vi "host.vi"() -> ()   [LabVIEW 2020]
uses:
  <vilib>/FPGAPlugInAG/cRIO-9035/niLvFpga_Open_cRIO-9035.vi
  <vilib>/rvi/interface/common/dynamic/niFpgaDynamicAddResources.vi
  <vilib>/Utility/error.llb/Error Cluster From Error Code.vi
  <vilib>/rvi/errors/niLvFpgaAdjustHostInterfaceError.vi
  <vilib>/FPGAPlugInAG/Dynamic/niLvFpga_Run_Dynamic.vi
  <vilib>/FPGAPlugInAG/Dynamic/niLvFpga_Close_Dynamic.vi
  <vilib>/rvi/interface/nirviOpenFPGA/nirviOpenFPGA.xnode
  FPGA Bitfiles/fftfpgaapplicati_FPGATarget_FFT2_NwCtSfbxiqQ.lvbitx
  FFT.vi
  <vilib>/rvi/interface/nirviMethod/nirviMethod.xnode
  <vilib>/rvi/interface/nirviCloseFPGA/nirviCloseFPGA.xnode
  <vilib>/rvi/errors/niLvFpgaMergeErrorWithErrorCode.vi
  <vilib>/FPGAPlugInAG/Dynamic/niLvFpga_ReadFifo_Dynamic.vi
  <vilib>/rvi/Analysis/host/Public/NI_FpgaMspHost.lvlib
  <vilib>/ptbypt/NI_PtbyPt.lvlib
  <vilib>/Analysis/NI_AALPro.lvlib
  <vilib>/FPGAPlugInAG/Dynamic/niLvFpga_WriteFifo_Dynamic.vi
panel:
  out "real size":i32
  out "img size":i32
  out "imaginary":dbl[](array[numeric])
  out "real":dbl[](array[numeric])
  out "imaginary number":dbl[](array[numeric])
  out "real number":dbl[](array[numeric])
  out "truth vs prediction vs error":dbl[][](graph)
  out "detrend acc":dbl[](graph)
  out "Array 3":dbl[](array[numeric])
  out "all rows":dbl[](array[numeric])
  out "XY Graph 2":cluster{dbl[], dbl[]}(graph)
  out "magnitude 2":dbl[](array[numeric])
  out "phase 2":dbl[](array[numeric])
  out "ploted signal from each selected frequency 2":dbl[][](graph)
  out "phase 1":dbl[](array[numeric])
  out "mag 1":dbl[](array[numeric])
  out "df (Hz) 2":dbl
  out "after FFT samples":i32
  out "xf (frequency)":dbl[](array[numeric])
  out "Before FFT samples":i32
  out "acc":dbl[](graph)
  out "samples":i32
  out "Array":fxp<+/-,32,16>[](array[numeric])
  out "end tick":fxp<+/-,32,16>[](array[numeric])
  out "start ticka":fxp<+/-,32,16>[](array[numeric])
  out "Waveform Graph":dbl[][](graph)
  out "input signal":T1(graph)
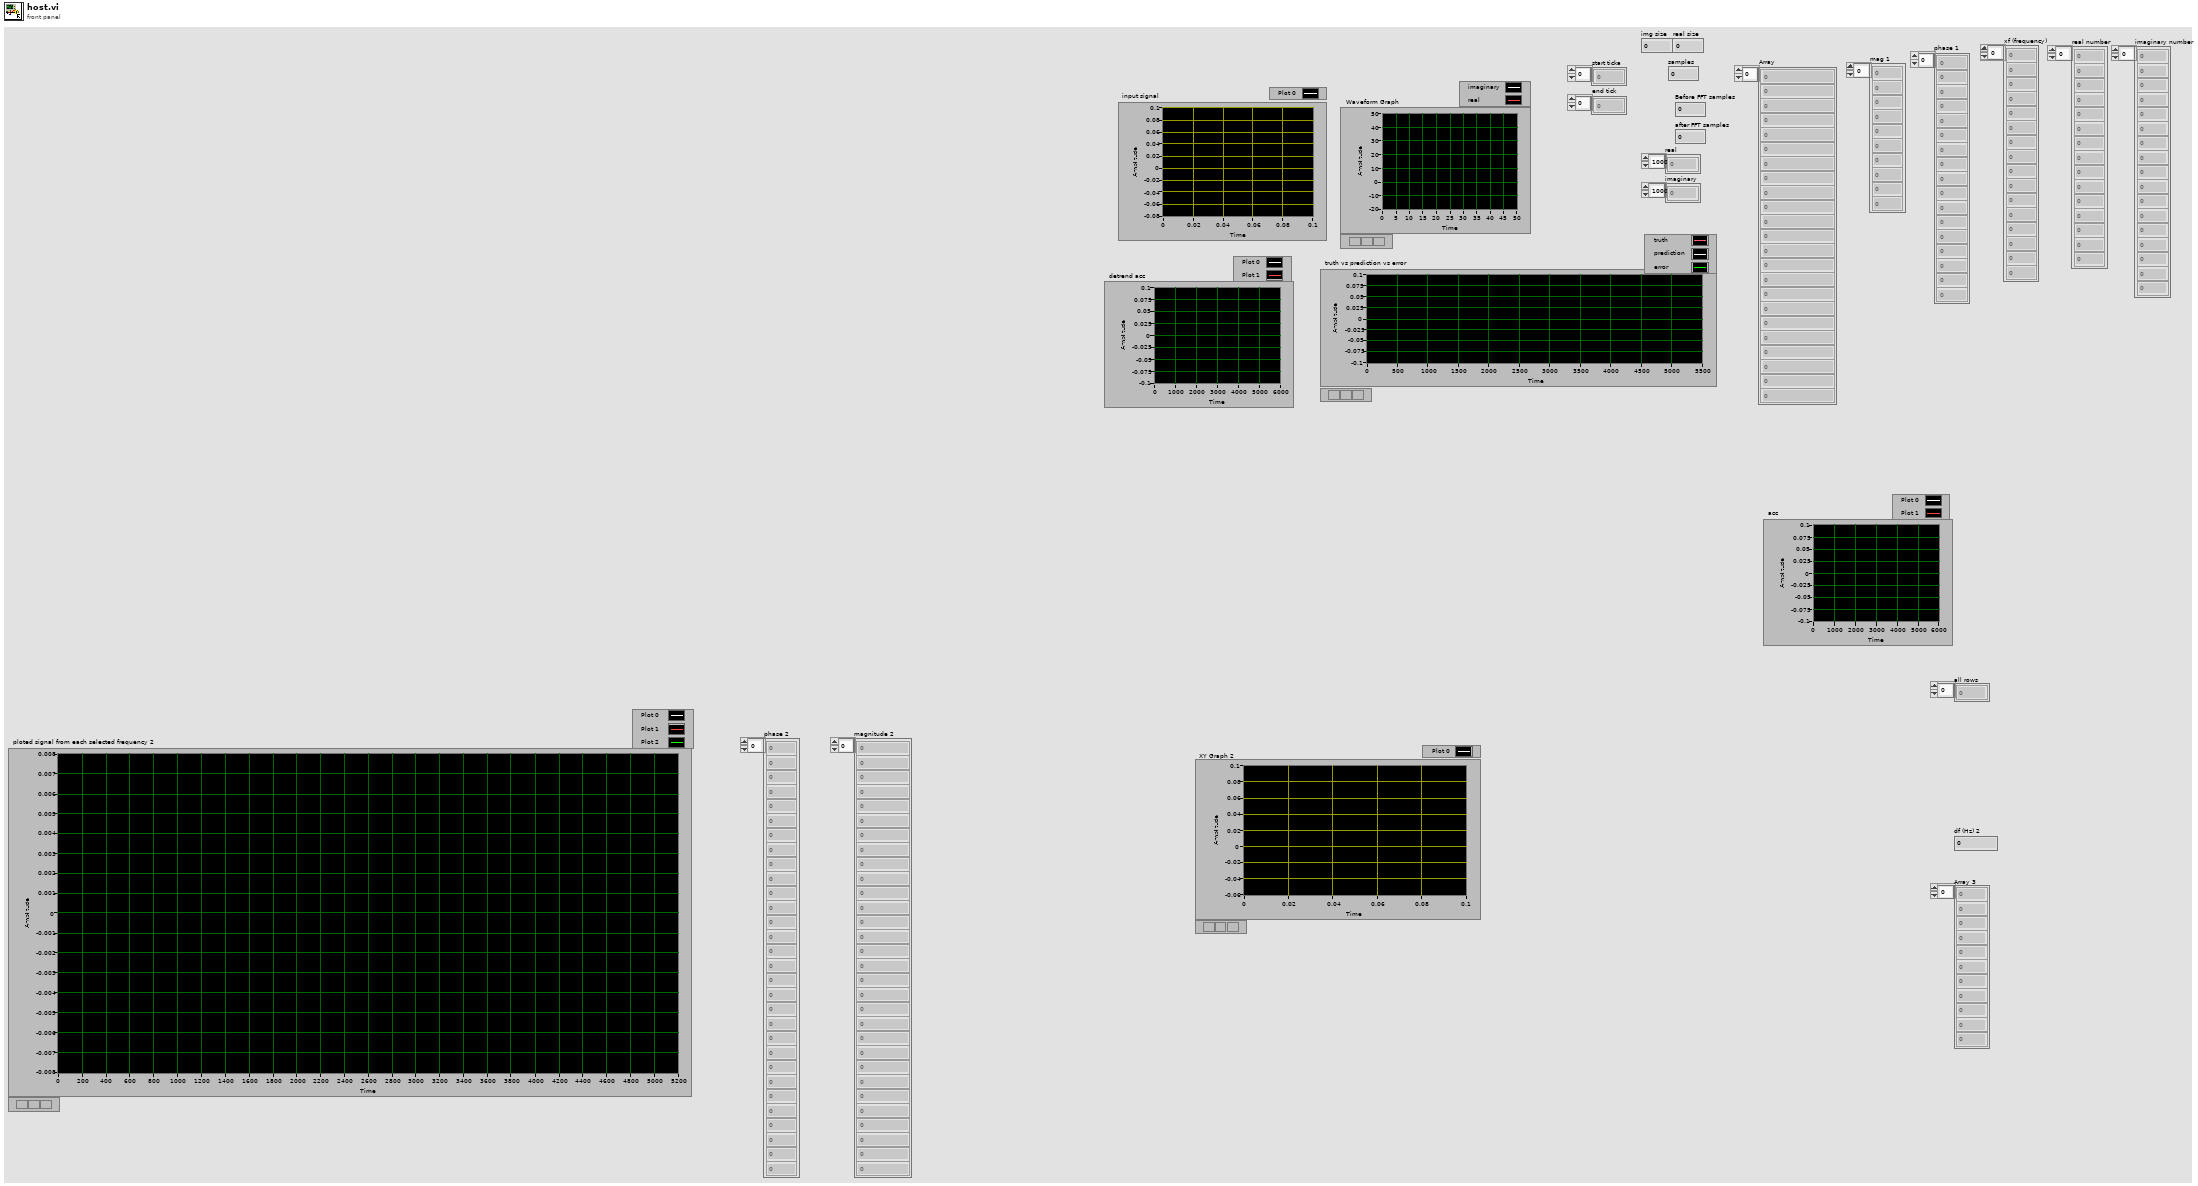
[diagram p1: front panel]
types:
  T1 = cluster{"array type (2D Dbl)":dbl[], "array type (2D Dbl)":dbl[]}
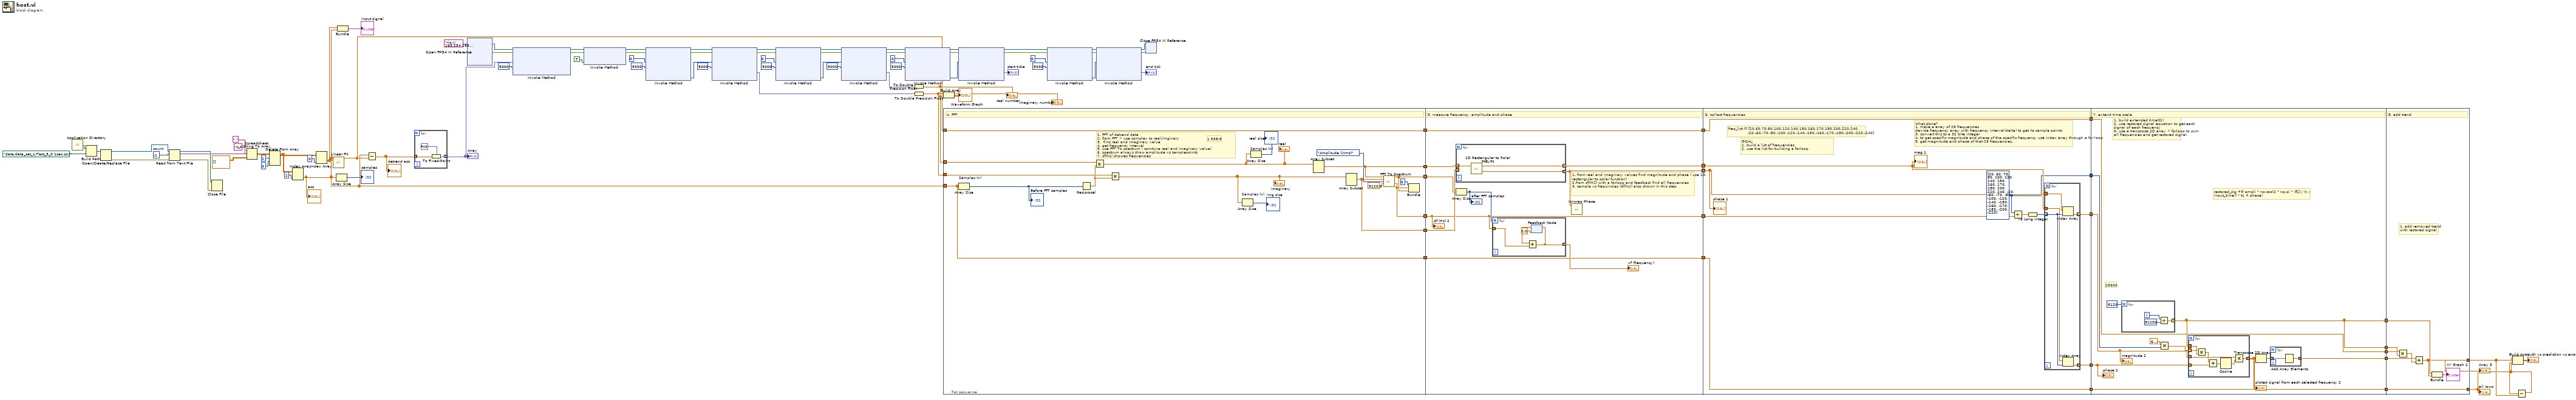
[diagram p0: block diagram]
diagram:
  w87 = -1  # count
  n1 = call <vilib>:"Application Directory.vi"() -> ("Application Directory"=w91:path)
  n2 = Build Path(base path=w91, name or relative path=path "data/data_set_1/Test_5_0.1sec.csv" ("default name")) -> (appended path=w90:path)
  n3 = Open/Create/Replace File(file path (use dialog)=w90) -> (refnum out=w95:refnum<file>, error out=w96:errorcluster)  [unwired: 5 in, 1 out]
  n4 = Read from Text File(file (use dialog)=w95, count=w87, error in=w96) -> (refnum out=w94:refnum<file>, text=w92:string, error out=w93:errorcluster)  [unwired: 1 in, 1 out]
  n5 = Close File(refnum=w94, error in=w93) -> ()  [unwired: 2 out]
  n6 = Spreadsheet String To Array(delimiter (Tab)=",", format string="%f", spreadsheet string=w92, array type (2D Dbl)=dbl[][] []) -> (array=w84:dbl[][])
  n7 = Delete From Array(array=w84, length=1, index (row)=0) -> (array with subset deleted=w79:dbl[][])  [unwired: 1 in, 1 out]
  n8 = Index Array(array=w79, index (col)=1 ("disabled index (col)")) -> (element=w6:dbl[])  [unwired: 1 in]
  "acc" <- w6
  n9 = Index Array(array=w79, index (col)=0 ("disabled index (col)")) -> (element=w10:dbl[])  [unwired: 1 in]
  n10 = call <vilib>:"Linear Fit.vi"("Y"=w6, "X"=w10) -> ("Best Linear Fit"=w7:dbl[])  [unwired: 9 in, 4 out]
  n11 = Array Size(array=w6) -> (size(s)=→"samples":i32)
  n12 = Bundle("array type (2D Dbl)"=w10, "array type (2D Dbl)"=w6) -> (→"input signal":T1)  [unwired: 1 in]
  n13 = Subtract(x=w6, y=w7) -> (x-y=w8:dbl[])
  "detrend acc" <- w8
  n14 = for {
    tunnel: [w98] -> w33 mode=indexing
    tunnel: w8 -> [w97] mode=indexing
    n15 = To Fixed-Point(fixed-point type=fxp<+/-,32,16> 0.0 ("f"), number=w97) -> (fixed-point=w98:fxp<+/-,32,16>)
  }
  "Array" <- w33
  n16 = xnode "Open FPGA VI Reference"("resource name"=tag "rio://169.254.183.73/RIO0") -> ("FPGA VI Reference Out"=w77:refnum<k20>, "error out"=w76:errorcluster)  [unwired: 1 in]
  n17 = xnode "Invoke Method"("FPGA VI Reference In"=w77, "error in"=w76, "Data"=w33, "Timeout (ms)"=5000) -> ("FPGA VI Reference Out"=w74:refnum<k20>, "error out"=w73:errorcluster)  [unwired: 1 out]
  n18 = xnode "Invoke Method"("FPGA VI Reference In"=w74, "error in"=w73, "Wait Until Done (F)"=TRUE) -> ("FPGA VI Reference Out"=w72:refnum<k20>, "error out"=w71:errorcluster)
  n19 = xnode "Invoke Method"("FPGA VI Reference In"=w72, "error in"=w71, "Number of Elements"=u32 0, "Timeout (ms)"=5000) -> ("FPGA VI Reference Out"=w70:refnum<k20>, "error out"=w69:errorcluster, "Elements Remaining"=w63:u32)  [unwired: 1 out]
  n20 = xnode "Invoke Method"("FPGA VI Reference In"=w70, "error in"=w69, "Number of Elements"=w63, "Timeout (ms)"=5000) -> ("FPGA VI Reference Out"=w66:refnum<k20>, "error out"=w65:errorcluster, "Data"=w60:fxp<+/-,32,16>[])  [unwired: 1 out]
  n21 = xnode "Invoke Method"("FPGA VI Reference In"=w66, "error in"=w65, "Number of Elements"=u32 0, "Timeout (ms)"=5000) -> ("FPGA VI Reference Out"=w68:refnum<k20>, "error out"=w67:errorcluster, "Elements Remaining"=w61:u32)  [unwired: 1 out]
  n22 = xnode "Invoke Method"("FPGA VI Reference In"=w68, "error in"=w67, "Number of Elements"=w61, "Timeout (ms)"=5000) -> ("FPGA VI Reference Out"=w56:refnum<k20>, "error out"=w55:errorcluster, "Data"=w59:fxp<+/-,32,16>[])  [unwired: 1 out]
  n23 = xnode "Invoke Method"("FPGA VI Reference In"=w56, "error in"=w55, "Number of Elements"=u32 0, "Timeout (ms)"=5000) -> ("FPGA VI Reference Out"=w54:refnum<k20>, "error out"=w53:errorcluster, "Elements Remaining"=w46:u32)  [unwired: 1 out]
  n24 = To Double Precision Float(number=w59) -> (double precision float=w5:dbl[])
  "real number" <- w5
  n25 = To Double Precision Float(number=w60) -> (double precision float=w9:dbl[])
  "imaginary number" <- w9
  n26 = Build Array(w9, w5) -> (→"Waveform Graph":dbl[][])
  n27 = flat-sequence {
    tunnel: [w115] -> w31
    tunnel: [w105] -> w30
    tunnel: [w104] -> w29
    tunnel: [w111] -> w28
    tunnel: [w110] -> w27
    tunnel: [w109] -> w26
    tunnel: w9 -> [w107]
    tunnel: w7 -> [w110]
    tunnel: w6 -> [w109]
    tunnel: w5 -> [w106]
    tunnel: w31 -> [w126]
    tunnel: w30 -> [w125]
    tunnel: w29 -> [w121]
    tunnel: w28 -> [w123]
    tunnel: [w121] -> w25
    tunnel: [w120] -> w24
    tunnel: [w119] -> w23
    tunnel: [w118] -> w22
    tunnel: w27 -> [w118]
    tunnel: w26 -> [w117]
    tunnel: [w117] -> w21
    tunnel: w25 -> [w135]
    tunnel: [w141] -> w20
    tunnel: w24 -> [w140]
    tunnel: w23 -> [w139]
    tunnel: [w138] -> w19
    tunnel: [w134] -> w18
    tunnel: [w137] -> w17
    tunnel: w22 -> [w137]
    tunnel: w21 -> [w136]
    tunnel: [w136] -> w16
    tunnel: w20 -> [w158]
    tunnel: w19 -> [w159]
    tunnel: w18 -> [w154]
    tunnel: [w152] -> w15
    tunnel: [w151] -> w14
    tunnel: w17 -> [w151]
    tunnel: [w150] -> w13
    tunnel: [w150] -> w12
    tunnel: w16 -> [w149]
    tunnel: [w149] -> w11
    tunnel: w15 -> [w181]
    tunnel: w14 -> [w179]
    tunnel: w13 -> [w180]
    tunnel: w12 -> [w178]
    tunnel: [w177] -> w2
    tunnel: w11 -> [w177]
    tunnel: [w176] -> w3
    frame #0 {
      # "1.95E-5"
      # "1. FFT of detrend data\n2. from FFT > use complex to real/imginary\n3.  find real and imaginary value\n4. get frequency interval\n5. use FFT To spectrum ( combine real and imaginary value)\n6. spectrum always show amplitude vs samplepoints\n7. df(hz) showes frequencies"
      # "4. FFT"
      n28 = Array Size "Samples (n)"(array=w109) -> (size(s)=w113:i32)
      "Before FFT samples" <- w113
      n29 = Reciprocal(x=w113) -> (1/x=w116:dbl)
      n30 = Multiply(x=w106, y=w116) -> (x*y=w101:dbl[])
      "real" <- w101
      n31 = Multiply(x=w107, y=w116) -> (x*y=w103:dbl[])
      "imaginary" <- w103
      n32 = Array Size "Samples (n)"(array=w103) -> (size(s)=→"img size":i32)
      n33 = Array Size "Samples (n)"(array=w101) -> (size(s)=→"real size":i32)
      n34 = Array Subset(array=w101) -> (w115:dbl[])  [unwired: 2 in]
      n35 = Array Subset(array=w103) -> (w105:dbl[])  [unwired: 2 in]
      n36 = call <vilib>:"FFT To Spectrum.vi"("real FFT data"=w115, "imaginary FFT data"=w105, "spectrum type"=enum8{"Power (Vrms^2)", "Amplitude (Vrms)"}."Amplitude (Vrms)", "sample rate (S/s)"=5120.0) -> ("spectrum out"=w111:dbl[], "df (Hz)"=w104:dbl)  [unwired: 9 in, 1 out]
      n37 = Bundle("index (row)"=0, "df (Hz)"=w104, "spectrum out"=w111) -> ()  [unwired: 1 in, 1 out]
    }
    frame #1 {
      # "1. from real and imaginary values find magnitude and phase ( use 1D rectangular to polar function)\n2.from df(HZ) with a forloop and feedback find all frequencies \n3. sample vs frequincies (df(hz)) also shown in this step"
      # "5. measure frequency, amplitude and phase"
      n38 = for {
        tunnel: w126 -> [w133] mode=indexing
        tunnel: w125 -> [_] mode=indexing
        tunnel: [w131] -> w120 mode=indexing
        tunnel: [w132] -> w119 mode=indexing
        n39 = call <vilib>:"1D Rectangular to Polar PtByPt.vi"("x"=w133) -> ("phase"=w132:dbl, "magnitude"=w131:dbl)  [unwired: 1 in]
      }
      n40 = Array Size(array=w123) -> (size(s)=w124:i32)
      "after FFT samples" <- w124
      n41 = for {
        N: w124 -> [_]
        tunnel: w121 -> [w129]
        tunnel: [w127] -> w122 mode=indexing
        n42 = feedback #1(0.0) -> (w130:dbl)
        n43 = Add(x=w130, y=w129) -> (x+y=w127:dbl)
        n44 = feedback-in #1(w127) -> ()
      }
      "xf (frequency)" <- w122
      n45 = call <vilib>:"Unwrap Phase.vi"("Phase"=w119) -> ()  [unwired: 9 in, 2 out]
      "df (Hz) 2" <- w121
    }
    frame #2 {
      w134 = i32[] [20, 60, 70, 80, 100, 120, 140, 150, 160, 170, 180, 200, 220, 240, -20, -60, -70, -80, -100, -120, -140, -150, -160, -170, -180, -200, -220]
      # "What done?\n1. make a array of 28 frequencies\ndevide frequency array with frequency interval(delta) to get its sample points\n3. convert this to a 32 bite integer\n4. to get specific magnitude and phase of the specific frequency use index array through a for loop\n5. get magnitude and phase of that 28 frequencies."
      # "freq_list = [20,60,70,80,100,120,140,150,160,170,180,200,220,240,\n                -20,-60,-70,-80,-100,-120,-140,-150,-160,-170,-180,-200,-220,-240]"
      # "GOAL:\n1. build a list of frequencies\n2. use the list for building a forloop"
      # "6. collect frequencies"
      n46 = Divide(x=w134, y=w135) -> (x/y=w143:dbl[])
      n47 = To Long Integer(number=w143) -> (32bit integer=w142:i32[])
      n48 = for {
        tunnel: w142 -> [w146] mode=indexing
        tunnel: w140 -> [w148]
        tunnel: [w147] -> w141 mode=indexing
        tunnel: w139 -> [w145]
        tunnel: [w144] -> w138 mode=indexing
        n49 = Index Array(array=w148, index=w146) -> (element=w147:dbl)
        n50 = Index Array(array=w145, index=w146) -> (element=w144:dbl)
      }
      "phase 1" <- w139
      "mag 1" <- w140
    }
    frame #3 {
      # "25600"
      # "1. build extended time(t1)\n2. use restored signal equation to get each signal of each frequency\n3. use a transpose 2D array > forloop to sum all frequencies and get restored signal."
      # "restored_sig += ampli * np.cos(2 * np.pi * (f[j] / (n / input_time)) * t1 + phase)"
      # "7. extend time scale"
      n51 = for {
        N: 5120 -> [_]
        tunnel: [w163] -> w150 mode=indexing
        i -> [w165]
        n52 = Divide(x=w165, y=51200) -> (x/y=w163:dbl)
      }
      n53 = Multiply(x=6.283185307179586, y=w154) -> (x*y=w153:dbl[])
      n54 = for {
        tunnel: w150 -> [w173]
        tunnel: w159 -> [w171] mode=indexing
        tunnel: w158 -> [w170] mode=indexing
        tunnel: [w169] -> w157 mode=indexing
        tunnel: w153 -> [w168] mode=indexing
        n55 = Multiply(x=w168, y=w173) -> (x*y=w172:dbl[])
        n56 = Add(x=w172, y=w171) -> (x+y=w167:dbl[])
        n57 = Cosine(x=w167) -> (cos(x)=w166:dbl[])
        n58 = Multiply(x=w170, y=w166) -> (x*y=w169:dbl[])
      }
      "ploted signal from each selected frequency 2" <- w157
      n59 = Transpose 2D Array(2D array=w157) -> (transposed array=w156:dbl[][])
      n60 = for {
        tunnel: w156 -> [w162] mode=indexing
        tunnel: [w161] -> w152 mode=indexing
        n61 = Add Array Elements(numeric array=w162) -> (sum=w161:dbl)
      }
      "magnitude 2" <- w158
      "phase 2" <- w159
    }
    frame #4 {
      # "1. add removed trend with restored signal"
      # "8. add trend"
      n62 = Multiply(x=w179, y=w178) -> (x*y=w174:dbl[])
      n63 = Add(x=w181, y=w174) -> (x+y=w176:dbl[])
      n64 = Bundle(w180, w176) -> (→"XY Graph 2":cluster{dbl[], dbl[]})  [unwired: 1 in]
    }
  }
  n65 = xnode "Invoke Method"("FPGA VI Reference In"=w54, "error in"=w53, "Number of Elements"=w46) -> ("FPGA VI Reference Out"=w52:refnum<k20>, "error out"=w51:errorcluster, "Data"=→"start ticka":fxp<+/-,32,16>[])  [unwired: 1 in, 1 out]
  n66 = xnode "Invoke Method"("FPGA VI Reference In"=w52, "error in"=w51, "Number of Elements"=u32 0, "Timeout (ms)"=5000) -> ("FPGA VI Reference Out"=w50:refnum<k20>, "error out"=w49:errorcluster, "Elements Remaining"=w44:u32)  [unwired: 1 out]
  n67 = xnode "Invoke Method"("FPGA VI Reference In"=w50, "error in"=w49, "Number of Elements"=w44) -> ("FPGA VI Reference Out"=w48:refnum<k20>, "error out"=w47:errorcluster, "Data"=→"end tick":fxp<+/-,32,16>[])  [unwired: 1 in, 1 out]
  n68 = xnode "Close FPGA VI Reference"("FPGA VI Reference In"=w48, "error in"=w47) -> ()  [unwired: 1 out]
  n69 = Subtract(x=w2, y=w3) -> (x-y=w1:dbl[])
  n70 = Build Array(w2, w3, w1) -> (→"truth vs prediction vs error":dbl[][])
  "all rows" <- w2
  "Array 3" <- w3
